vi "Poly_SetPWM.vi"   [LabVIEW 2012]
doc: "Creates a PWM output through the specified \"Port\" according to the specified value of \"Variable in\"."
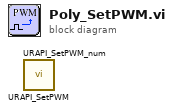
[diagram p0: block diagram]
diagram:
  n1 = call <userlib>:"URAPI_SetPWM.vi"() -> ()  [unwired: 4 in, 2 out]
  n2 = call <userlib>:"URAPI_SetPWM_num.vi"() -> ()  [unwired: 4 in, 2 out]
